vi "GAME.vi"() -> ()   [LabVIEW 2014]
panel:
  out "output 2":string[][](array[string])
  in  "8 8":string
  in  "8 7":string
  in  "8 6":string
  in  "8 5":string="7"
  in  "8 4":string
  in  "8 3":string
  in  "8 2":string
  in  "8 1":string="5"
  in  "8 0":string
  in  "7 3":string="6"
  in  "6 3":string
  in  "5 3":string="8"
  in  "4 3":string
  in  "3 2":string
  in  "2 4":string="2"
  in  "1 1":string="2"
  in  "0 8":string
  in  "0 0":string
  in  "7 8":string
  in  "7 7":string="5"
  in  "7 6":string
  in  "7 5":string
  in  "7 4":string="9"
  in  "6 8":string
  in  "6 7":string
  in  "6 6":string="8"
  in  "6 5":string
  in  "6 4":string="5"
  in  "5 8":string
  in  "5 7":string="2"
  in  "5 6":string
  in  "5 5":string
  in  "5 4":string
  in  "4 8":string="1"
  in  "4 7":string
  in  "4 6":string="3"
  in  "4 5":string
  in  "4 4":string
  in  "3 8":string
  in  "3 7":string
  in  "3 6":string
  in  "3 5":string="3"
  in  "3 4":string
  in  "3 3":string
  in  "2 8":string="5"
  in  "2 7":string
  in  "2 6":string="4"
  in  "2 5":string
  in  "1 8":string="8"
  in  "1 7":string
  in  "1 6":string
  in  "1 5":string="4"
  in  "1 4":string="3"
  in  "1 3":string
  in  "1 2":string
  in  "0 7":string="7"
  in  "0 6":string
  in  "0 5":string
  in  "0 4":string="5"
  in  "0 3":string
  in  "0 2":string
  in  "0 1":string
  in  "7 2":string
  in  "7 1":string
  in  "7 0":string="8"
  in  "6 2":string="4"
  in  "6 1":string
  in  "6 0":string="9"
  in  "5 2":string
  in  "5 1":string
  in  "5 0":string
  in  "4 2":string="9"
  in  "4 1":string
  in  "4 0":string="6"
  in  "3 1":string="7"
  in  "3 0":string
  in  "2 3":string
  in  "2 2":string="1"
  in  "2 1":string
  in  "2 0":string
  in  "1 0":string
  in  "stop":bool
  # "SUDOKU"
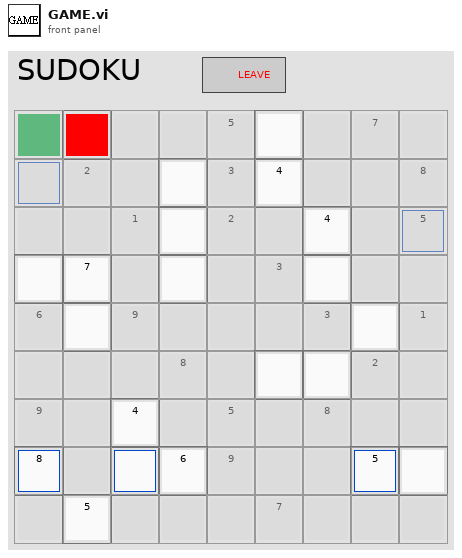
[diagram p1: front panel]
types:
  T1 = enum8{"Enabled", "Disabled", "Disabled and Grayed Out"}
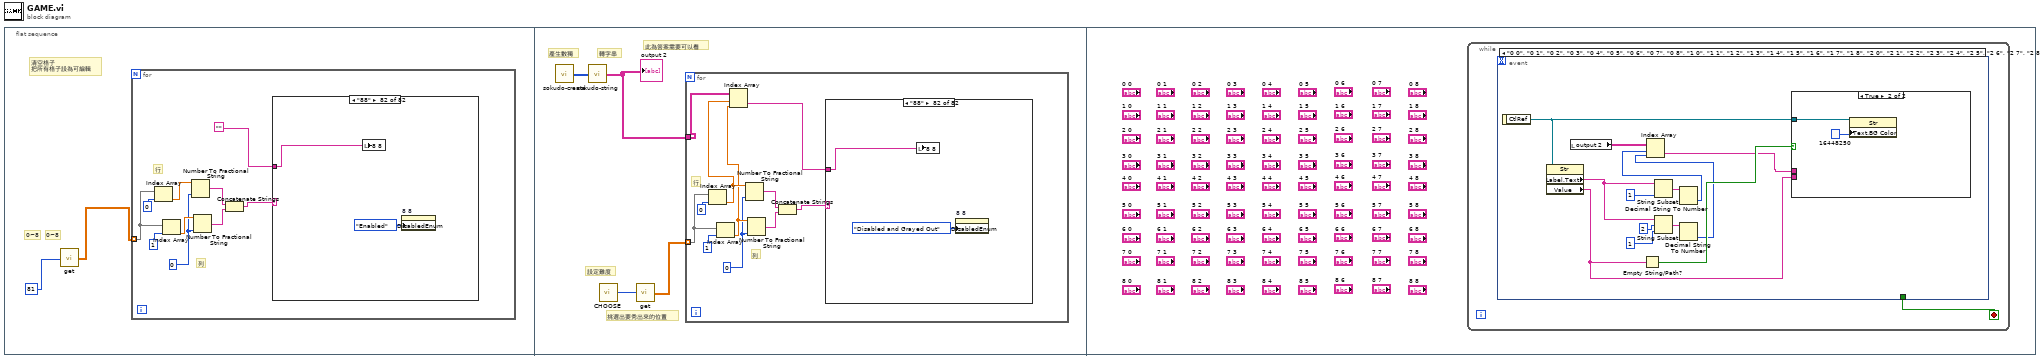
[diagram p0: block diagram]
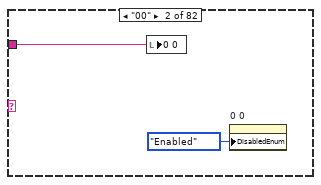
[diagram p3: hidden frame]
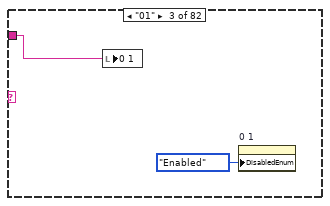
[diagram p4: hidden frame]
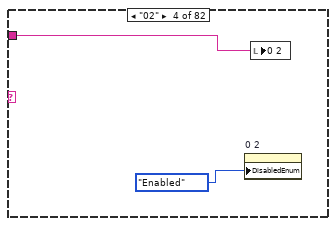
[diagram p5: hidden frame]
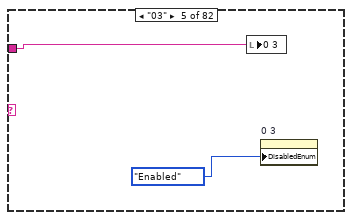
[diagram p6: hidden frame]
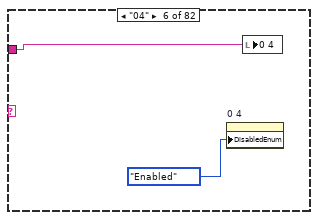
[diagram p7: hidden frame]
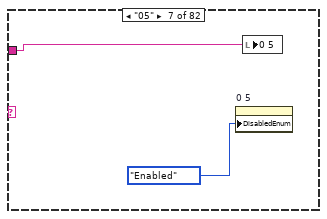
[diagram p8: hidden frame]
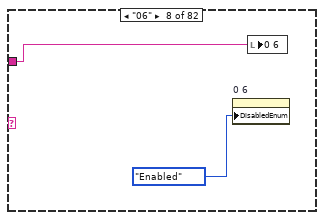
[diagram p9: hidden frame]
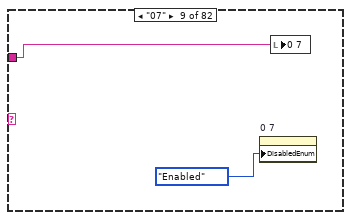
[diagram p10: hidden frame]
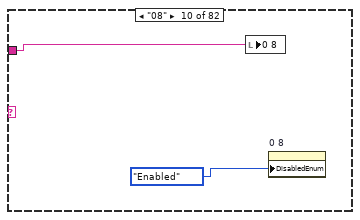
[diagram p11: hidden frame]
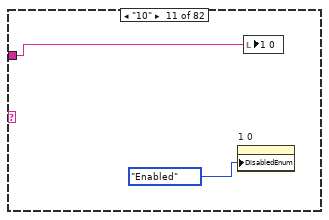
[diagram p12: hidden frame]
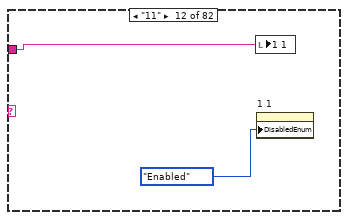
[diagram p13: hidden frame]
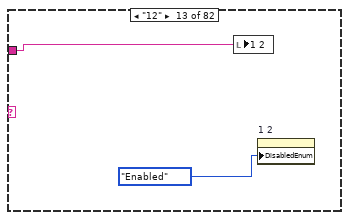
[diagram p14: hidden frame]
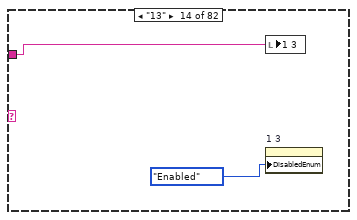
[diagram p15: hidden frame]
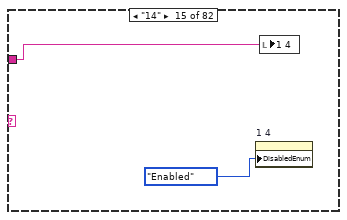
[diagram p16: hidden frame]
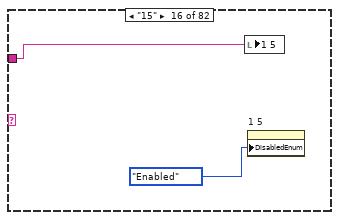
[diagram p17: hidden frame]
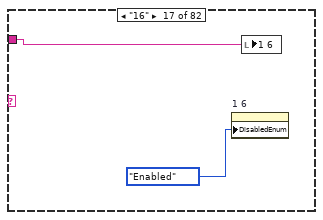
[diagram p18: hidden frame]
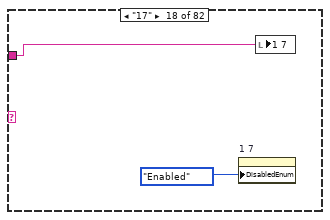
[diagram p19: hidden frame]
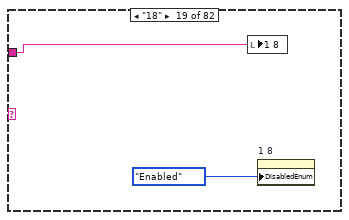
[diagram p20: hidden frame]
diagram:
  n1 = flat-sequence {
    frame #0 {
      # "0~8"
      # "0~8"
      # "清空格子\n把所有格子設為可編輯"
      n2 = call "get.vi"("Numeric 2"=81) -> ("SHOW"=w2:dbl[][])
      n3 = for {
        tunnel: w2 -> [w11] mode=indexing
        w5 = 0
        # "列"
        # "行"
        n4 = Index Array(array=w11, index=0) -> (element=w7:dbl)
        n5 = Index Array(array=w11, index=1) -> (element=w6:dbl)
        n6 = Number To Fractional String(number=w7, precision (6)=w5) -> (F-format string=w9:string)  [unwired: 2 in]
        n7 = Number To Fractional String(number=w6, precision (6)=w5) -> (F-format string=w8:string)  [unwired: 2 in]
        n8 = Concatenate Strings(w9, w8) -> (w4:string)
        n9 = case shown="\"88\"" w4 {
          tunnel: "" -> [_ w14 w16 w18 w20 w22 w24 w26 w28 w30 w32 w34 w36 w38 w40 w42 w44 w46 w48 w50 w52 w54 w56 w58 w60 w62 w64 w66 w68 w70 w72 w74 w76 w78 w80 w82 w84 w86 w88 w90 w92 w94 w96 w98 w100 w102 w104 w106 w108 w110 w112 w114 w116 w118 w120 w122 w124 w126 w128 w130 w132 w134 w136 w138 w140 w142 w144 w146 w148 w150 w152 w154 w156 w158 w160 w162 w164 w166 w168 w170 w172 w174]
          frame "False", Default {
          }
          frame "00" {
            n10 = local write "0 0"(w14) -> ()
            n11 = property on="0 0" class="Str"("DisabledEnum"=T1."Enabled" ("Disabled")) -> ()  [unwired: 2 in, 2 out]
          }
          frame "01" {
            n12 = local write "0 1"(w16) -> ()
            n13 = property on="0 1" class="Str"("DisabledEnum"=T1."Enabled" ("Disabled")) -> ()  [unwired: 2 in, 2 out]
          }
          frame "02" {
            n14 = property on="0 2" class="Str"("DisabledEnum"=T1."Enabled" ("Disabled")) -> ()  [unwired: 2 in, 2 out]
            n15 = local write "0 2"(w18) -> ()
          }
          frame "03" {
            n16 = local write "0 3"(w20) -> ()
            n17 = property on="0 3" class="Str"("DisabledEnum"=T1."Enabled" ("Disabled")) -> ()  [unwired: 2 in, 2 out]
          }
          frame "04" {
            n18 = property on="0 4" class="Str"("DisabledEnum"=T1."Enabled" ("Disabled")) -> ()  [unwired: 2 in, 2 out]
            n19 = local write "0 4"(w22) -> ()
          }
          frame "05" {
            n20 = property on="0 5" class="Str"("DisabledEnum"=T1."Enabled" ("Disabled")) -> ()  [unwired: 2 in, 2 out]
            n21 = local write "0 5"(w24) -> ()
          }
          frame "06" {
            n22 = property on="0 6" class="Str"("DisabledEnum"=T1."Enabled" ("Disabled")) -> ()  [unwired: 2 in, 2 out]
            n23 = local write "0 6"(w26) -> ()
          }
          frame "07" {
            n24 = property on="0 7" class="Str"("DisabledEnum"=T1."Enabled" ("Disabled")) -> ()  [unwired: 2 in, 2 out]
            n25 = local write "0 7"(w28) -> ()
          }
          frame "08" {
            n26 = local write "0 8"(w30) -> ()
            n27 = property on="0 8" class="Str"("DisabledEnum"=T1."Enabled" ("Disabled")) -> ()  [unwired: 2 in, 2 out]
          }
          frame "10" {
            n28 = property on="1 0" class="Str"("DisabledEnum"=T1."Enabled" ("Disabled")) -> ()  [unwired: 2 in, 2 out]
            n29 = local write "1 0"(w32) -> ()
          }
          frame "11" {
            n30 = local write "1 1"(w34) -> ()
            n31 = property on="1 1" class="Str"("DisabledEnum"=T1."Enabled" ("Disabled")) -> ()  [unwired: 2 in, 2 out]
          }
          frame "12" {
            n32 = local write "1 2"(w36) -> ()
            n33 = property on="1 2" class="Str"("DisabledEnum"=T1."Enabled" ("Disabled")) -> ()  [unwired: 2 in, 2 out]
          }
          frame "13" {
            n34 = local write "1 3"(w38) -> ()
            n35 = property on="1 3" class="Str"("DisabledEnum"=T1."Enabled" ("Disabled")) -> ()  [unwired: 2 in, 2 out]
          }
          frame "14" {
            n36 = property on="1 4" class="Str"("DisabledEnum"=T1."Enabled" ("Disabled")) -> ()  [unwired: 2 in, 2 out]
            n37 = local write "1 4"(w40) -> ()
          }
          frame "15" {
            n38 = local write "1 5"(w42) -> ()
            n39 = property on="1 5" class="Str"("DisabledEnum"=T1."Enabled" ("Disabled")) -> ()  [unwired: 2 in, 2 out]
          }
          frame "16" {
            n40 = property on="1 6" class="Str"("DisabledEnum"=T1."Enabled" ("Disabled")) -> ()  [unwired: 2 in, 2 out]
            n41 = local write "1 6"(w44) -> ()
          }
          frame "17" {
            n42 = property on="1 7" class="Str"("DisabledEnum"=T1."Enabled" ("Disabled")) -> ()  [unwired: 2 in, 2 out]
            n43 = local write "1 7"(w46) -> ()
          }
          frame "18" {
            n44 = local write "1 8"(w48) -> ()
            n45 = property on="1 8" class="Str"("DisabledEnum"=T1."Enabled" ("Disabled")) -> ()  [unwired: 2 in, 2 out]
          }
          frame "20" {
            n46 = local write "2 0"(w50) -> ()
            n47 = property on="2 0" class="Str"("DisabledEnum"=T1."Enabled" ("Disabled")) -> ()  [unwired: 2 in, 2 out]
          }
          frame "21" {
            n48 = local write "2 1"(w52) -> ()
            n49 = property on="2 1" class="Str"("DisabledEnum"=T1."Enabled" ("Disabled")) -> ()  [unwired: 2 in, 2 out]
          }
          frame "22" {
            n50 = local write "2 2"(w54) -> ()
            n51 = property on="2 2" class="Str"("DisabledEnum"=T1."Enabled" ("Disabled")) -> ()  [unwired: 2 in, 2 out]
          }
          frame "23" {
            n52 = local write "2 3"(w56) -> ()
            n53 = property on="2 3" class="Str"("DisabledEnum"=T1."Enabled" ("Disabled")) -> ()  [unwired: 2 in, 2 out]
          }
          frame "24" {
            n54 = property on="2 4" class="Str"("DisabledEnum"=T1."Enabled" ("Disabled")) -> ()  [unwired: 2 in, 2 out]
            n55 = local write "2 4"(w58) -> ()
          }
          frame "25" {
            n56 = local write "2 5"(w60) -> ()
            n57 = property on="2 5" class="Str"("DisabledEnum"=T1."Enabled" ("Disabled")) -> ()  [unwired: 2 in, 2 out]
          }
          frame "26" {
            n58 = local write "2 6"(w62) -> ()
            n59 = property on="2 6" class="Str"("DisabledEnum"=T1."Enabled" ("Disabled")) -> ()  [unwired: 2 in, 2 out]
          }
          frame "27" {
            n60 = property on="2 7" class="Str"("DisabledEnum"=T1."Enabled" ("Disabled")) -> ()  [unwired: 2 in, 2 out]
            n61 = local write "2 7"(w64) -> ()
          }
          frame "28" {
            n62 = property on="2 8" class="Str"("DisabledEnum"=T1."Enabled" ("Disabled")) -> ()  [unwired: 2 in, 2 out]
            n63 = local write "2 8"(w66) -> ()
          }
          frame "30" {
            n64 = property on="3 0" class="Str"("DisabledEnum"=T1."Enabled" ("Disabled")) -> ()  [unwired: 2 in, 2 out]
            n65 = local write "3 0"(w68) -> ()
          }
          frame "31" {
            n66 = local write "3 1"(w70) -> ()
            n67 = property on="3 1" class="Str"("DisabledEnum"=T1."Enabled" ("Disabled")) -> ()  [unwired: 2 in, 2 out]
          }
          frame "32" {
            n68 = local write "3 2"(w72) -> ()
            n69 = property on="3 2" class="Str"("DisabledEnum"=T1."Enabled" ("Disabled")) -> ()  [unwired: 2 in, 2 out]
          }
          frame "33" {
            n70 = local write "3 3"(w74) -> ()
            n71 = property on="3 3" class="Str"("DisabledEnum"=T1."Enabled" ("Disabled")) -> ()  [unwired: 2 in, 2 out]
          }
          frame "34" {
            n72 = local write "3 4"(w76) -> ()
            n73 = property on="3 4" class="Str"("DisabledEnum"=T1."Enabled" ("Disabled")) -> ()  [unwired: 2 in, 2 out]
          }
          frame "35" {
            n74 = property on="3 5" class="Str"("DisabledEnum"=T1."Enabled" ("Disabled")) -> ()  [unwired: 2 in, 2 out]
            n75 = local write "3 5"(w78) -> ()
          }
          frame "36" {
            n76 = local write "3 6"(w80) -> ()
            n77 = property on="3 6" class="Str"("DisabledEnum"=T1."Enabled" ("Disabled")) -> ()  [unwired: 2 in, 2 out]
          }
          frame "37" {
            n78 = property on="3 7" class="Str"("DisabledEnum"=T1."Enabled" ("Disabled")) -> ()  [unwired: 2 in, 2 out]
            n79 = local write "3 7"(w82) -> ()
          }
          frame "38" {
            n80 = property on="3 8" class="Str"("DisabledEnum"=T1."Enabled" ("Disabled")) -> ()  [unwired: 2 in, 2 out]
            n81 = local write "3 8"(w84) -> ()
          }
          frame "40" {
            n82 = local write "4 0"(w86) -> ()
            n83 = property on="4 0" class="Str"("DisabledEnum"=T1."Enabled" ("Disabled")) -> ()  [unwired: 2 in, 2 out]
          }
          frame "41" {
            n84 = property on="4 1" class="Str"("DisabledEnum"=T1."Enabled" ("Disabled")) -> ()  [unwired: 2 in, 2 out]
            n85 = local write "4 1"(w88) -> ()
          }
          frame "42" {
            n86 = local write "4 2"(w90) -> ()
            n87 = property on="4 2" class="Str"("DisabledEnum"=T1."Enabled" ("Disabled")) -> ()  [unwired: 2 in, 2 out]
          }
          frame "43" {
            n88 = property on="4 3" class="Str"("DisabledEnum"=T1."Enabled" ("Disabled")) -> ()  [unwired: 2 in, 2 out]
            n89 = local write "4 3"(w92) -> ()
          }
          frame "44" {
            n90 = local write "4 4"(w94) -> ()
            n91 = property on="4 4" class="Str"("DisabledEnum"=T1."Enabled" ("Disabled")) -> ()  [unwired: 2 in, 2 out]
          }
          frame "45" {
            n92 = local write "4 5"(w96) -> ()
            n93 = property on="4 5" class="Str"("DisabledEnum"=T1."Enabled" ("Disabled")) -> ()  [unwired: 2 in, 2 out]
          }
          frame "46" {
            n94 = local write "4 6"(w98) -> ()
            n95 = property on="4 6" class="Str"("DisabledEnum"=T1."Enabled" ("Disabled")) -> ()  [unwired: 2 in, 2 out]
          }
          frame "47" {
            n96 = local write "4 7"(w100) -> ()
            n97 = property on="4 7" class="Str"("DisabledEnum"=T1."Enabled" ("Disabled")) -> ()  [unwired: 2 in, 2 out]
          }
          frame "48" {
            n98 = local write "4 8"(w102) -> ()
            n99 = property on="4 8" class="Str"("DisabledEnum"=T1."Enabled" ("Disabled")) -> ()  [unwired: 2 in, 2 out]
          }
          frame "50" {
            n100 = local write "5 0"(w104) -> ()
            n101 = property on="5 0" class="Str"("DisabledEnum"=T1."Enabled" ("Disabled")) -> ()  [unwired: 2 in, 2 out]
          }
          frame "51" {
            n102 = local write "5 1"(w106) -> ()
            n103 = property on="5 1" class="Str"("DisabledEnum"=T1."Enabled" ("Disabled")) -> ()  [unwired: 2 in, 2 out]
          }
          frame "52" {
            n104 = property on="5 2" class="Str"("DisabledEnum"=T1."Enabled" ("Disabled")) -> ()  [unwired: 2 in, 2 out]
            n105 = local write "5 2"(w108) -> ()
          }
          frame "53" {
            n106 = local write "5 3"(w110) -> ()
            n107 = property on="5 3" class="Str"("DisabledEnum"=T1."Enabled" ("Disabled")) -> ()  [unwired: 2 in, 2 out]
          }
          frame "54" {
            n108 = local write "5 4"(w112) -> ()
            n109 = property on="5 4" class="Str"("DisabledEnum"=T1."Enabled" ("Disabled")) -> ()  [unwired: 2 in, 2 out]
          }
          frame "55" {
            n110 = local write "5 5"(w114) -> ()
            n111 = property on="5 5" class="Str"("DisabledEnum"=T1."Enabled" ("Disabled")) -> ()  [unwired: 2 in, 2 out]
          }
          frame "56" {
            n112 = property on="5 6" class="Str"("DisabledEnum"=T1."Enabled" ("Disabled")) -> ()  [unwired: 2 in, 2 out]
            n113 = local write "5 6"(w116) -> ()
          }
          frame "57" {
            n114 = local write "5 7"(w118) -> ()
            n115 = property on="5 7" class="Str"("DisabledEnum"=T1."Enabled" ("Disabled")) -> ()  [unwired: 2 in, 2 out]
          }
          frame "58" {
            n116 = property on="5 8" class="Str"("DisabledEnum"=T1."Enabled" ("Disabled")) -> ()  [unwired: 2 in, 2 out]
            n117 = local write "5 8"(w120) -> ()
          }
          frame "60" {
            n118 = local write "6 0"(w122) -> ()
            n119 = property on="6 0" class="Str"("DisabledEnum"=T1."Enabled" ("Disabled")) -> ()  [unwired: 2 in, 2 out]
          }
          frame "61" {
            n120 = local write "6 1"(w124) -> ()
            n121 = property on="6 1" class="Str"("DisabledEnum"=T1."Enabled" ("Disabled")) -> ()  [unwired: 2 in, 2 out]
          }
          frame "62" {
            n122 = local write "6 2"(w126) -> ()
            n123 = property on="6 2" class="Str"("DisabledEnum"=T1."Enabled" ("Disabled")) -> ()  [unwired: 2 in, 2 out]
          }
          frame "63" {
            n124 = local write "6 3"(w128) -> ()
            n125 = property on="6 3" class="Str"("DisabledEnum"=T1."Enabled" ("Disabled")) -> ()  [unwired: 2 in, 2 out]
          }
          frame "64" {
            n126 = local write "6 4"(w130) -> ()
            n127 = property on="6 4" class="Str"("DisabledEnum"=T1."Enabled" ("Disabled")) -> ()  [unwired: 2 in, 2 out]
          }
          frame "65" {
            n128 = local write "6 5"(w132) -> ()
            n129 = property on="6 5" class="Str"("DisabledEnum"=T1."Enabled" ("Disabled")) -> ()  [unwired: 2 in, 2 out]
          }
          frame "66" {
            n130 = property on="6 6" class="Str"("DisabledEnum"=T1."Enabled" ("Disabled")) -> ()  [unwired: 2 in, 2 out]
            n131 = local write "6 6"(w134) -> ()
          }
          frame "67" {
            n132 = property on="6 7" class="Str"("DisabledEnum"=T1."Enabled" ("Disabled")) -> ()  [unwired: 2 in, 2 out]
            n133 = local write "6 7"(w136) -> ()
          }
          frame "68" {
            n134 = local write "6 8"(w138) -> ()
            n135 = property on="6 8" class="Str"("DisabledEnum"=T1."Enabled" ("Disabled")) -> ()  [unwired: 2 in, 2 out]
          }
          frame "70" {
            n136 = property on="7 0" class="Str"("DisabledEnum"=T1."Enabled" ("Disabled")) -> ()  [unwired: 2 in, 2 out]
            n137 = local write "7 0"(w140) -> ()
          }
          frame "71" {
            n138 = property on="7 1" class="Str"("DisabledEnum"=T1."Enabled" ("Disabled")) -> ()  [unwired: 2 in, 2 out]
            n139 = local write "7 1"(w142) -> ()
          }
          frame "72" {
            n140 = local write "7 2"(w144) -> ()
            n141 = property on="7 2" class="Str"("DisabledEnum"=T1."Enabled" ("Disabled")) -> ()  [unwired: 2 in, 2 out]
          }
          frame "73" {
            n142 = local write "7 3"(w146) -> ()
            n143 = property on="7 3" class="Str"("DisabledEnum"=T1."Enabled" ("Disabled")) -> ()  [unwired: 2 in, 2 out]
          }
          frame "74" {
            n144 = property on="7 4" class="Str"("DisabledEnum"=T1."Enabled" ("Disabled")) -> ()  [unwired: 2 in, 2 out]
            n145 = local write "7 4"(w148) -> ()
          }
          frame "75" {
            n146 = local write "7 5"(w150) -> ()
            n147 = property on="7 5" class="Str"("DisabledEnum"=T1."Enabled" ("Disabled")) -> ()  [unwired: 2 in, 2 out]
          }
          frame "76" {
            n148 = property on="7 6" class="Str"("DisabledEnum"=T1."Enabled" ("Disabled")) -> ()  [unwired: 2 in, 2 out]
            n149 = local write "7 6"(w152) -> ()
          }
          frame "77" {
            n150 = local write "7 7"(w154) -> ()
            n151 = property on="7 7" class="Str"("DisabledEnum"=T1."Enabled" ("Disabled")) -> ()  [unwired: 2 in, 2 out]
          }
          frame "78" {
            n152 = property on="7 8" class="Str"("DisabledEnum"=T1."Enabled" ("Disabled")) -> ()  [unwired: 2 in, 2 out]
            n153 = local write "7 8"(w156) -> ()
          }
          frame "80" {
            n154 = property on="8 0" class="Str"("DisabledEnum"=T1."Enabled" ("Disabled")) -> ()  [unwired: 2 in, 2 out]
            n155 = local write "8 0"(w158) -> ()
          }
          frame "81" {
            n156 = local write "8 1"(w160) -> ()
            n157 = property on="8 1" class="Str"("DisabledEnum"=T1."Enabled" ("Disabled")) -> ()  [unwired: 2 in, 2 out]
          }
          frame "82" {
            n158 = local write "8 2"(w162) -> ()
            n159 = property on="8 2" class="Str"("DisabledEnum"=T1."Enabled" ("Disabled")) -> ()  [unwired: 2 in, 2 out]
          }
          frame "83" {
            n160 = local write "8 3"(w164) -> ()
            n161 = property on="8 3" class="Str"("DisabledEnum"=T1."Enabled" ("Disabled")) -> ()  [unwired: 2 in, 2 out]
          }
          frame "84" {
            n162 = local write "8 4"(w166) -> ()
            n163 = property on="8 4" class="Str"("DisabledEnum"=T1."Enabled" ("Disabled")) -> ()  [unwired: 2 in, 2 out]
          }
          frame "85" {
            n164 = local write "8 5"(w168) -> ()
            n165 = property on="8 5" class="Str"("DisabledEnum"=T1."Enabled" ("Disabled")) -> ()  [unwired: 2 in, 2 out]
          }
          frame "86" {
            n166 = property on="8 6" class="Str"("DisabledEnum"=T1."Enabled" ("Disabled")) -> ()  [unwired: 2 in, 2 out]
            n167 = local write "8 6"(w170) -> ()
          }
          frame "87" {
            n168 = local write "8 7"(w172) -> ()
            n169 = property on="8 7" class="Str"("DisabledEnum"=T1."Enabled" ("Disabled")) -> ()  [unwired: 2 in, 2 out]
          }
          frame "88" {
            n170 = local write "8 8"(w174) -> ()
            n171 = property on="8 8" class="Str"("DisabledEnum"=T1."Enabled" ("Disabled")) -> ()  [unwired: 2 in, 2 out]
          }
        }
      }
    }
    frame #1 {
      # "轉字串"
      # "挑選出要秀出來的位置"
      # "設定難度"
      # "產生數獨"
      # "此為答案需要可以看"
      n172 = call "sokudo-create.vi"() -> ("Sudoku"=w178:i32[][])  [unwired: 1 in]
      n173 = call "sokudo-string.vi"("Input"=w178) -> ("output"=w177:string[][])
      "output 2" <- w177
      n174 = call "CHOOSE.vi"() -> ("Numeric"=w176:i32)  [unwired: 1 in]
      n175 = call "get.vi"("Numeric 2"=w176) -> ("SHOW"=w175:dbl[][])
      n176 = for {
        tunnel: w175 -> [w188] mode=indexing
        tunnel: w177 -> [w184]
        w180 = 0
        # "列"
        # "行"
        n177 = Index Array(array=w188, index=0) -> (element=w182:dbl)
        n178 = Index Array(array=w188, index=1) -> (element=w181:dbl)
        n179 = Index Array(array=w184, index (row)=w182, index (col)=w181) -> (element=w183:string)
        n180 = Number To Fractional String(number=w182, precision (6)=w180) -> (F-format string=w186:string)  [unwired: 2 in]
        n181 = Number To Fractional String(number=w181, precision (6)=w180) -> (F-format string=w185:string)  [unwired: 2 in]
        n182 = Concatenate Strings(w186, w185) -> (w179:string)
        n183 = case shown="\"88\"" w179 {
          tunnel: w183 -> [_ w191 w193 w195 w197 w199 w201 w203 w205 w207 w209 w211 w213 w215 w217 w219 w221 w223 w225 w227 w229 w231 w233 w235 w237 w239 w241 w243 w245 w247 w249 w251 w253 w255 w257 w259 w261 w263 w265 w267 w269 w271 w273 w275 w277 w279 w281 w283 w285 w287 w289 w291 w293 w295 w297 w299 w301 w303 w305 w307 w309 w311 w313 w315 w317 w319 w321 w323 w325 w327 w329 w331 w333 w335 w337 w339 w341 w343 w345 w347 w349 w351]
          frame "False", Default {
          }
          frame "00" {
            n184 = local write "0 0"(w191) -> ()
            n185 = property on="0 0" class="Str"("DisabledEnum"=T1."Disabled and Grayed Out" ("Disabled")) -> ()  [unwired: 2 in, 2 out]
          }
          frame "01" {
            n186 = local write "0 1"(w193) -> ()
            n187 = property on="0 1" class="Str"("DisabledEnum"=T1."Disabled and Grayed Out" ("Disabled")) -> ()  [unwired: 2 in, 2 out]
          }
          frame "02" {
            n188 = property on="0 2" class="Str"("DisabledEnum"=T1."Disabled and Grayed Out" ("Disabled")) -> ()  [unwired: 2 in, 2 out]
            n189 = local write "0 2"(w195) -> ()
          }
          frame "03" {
            n190 = local write "0 3"(w197) -> ()
            n191 = property on="0 3" class="Str"("DisabledEnum"=T1."Disabled and Grayed Out" ("Disabled")) -> ()  [unwired: 2 in, 2 out]
          }
          frame "04" {
            n192 = property on="0 4" class="Str"("DisabledEnum"=T1."Disabled and Grayed Out" ("Disabled")) -> ()  [unwired: 2 in, 2 out]
            n193 = local write "0 4"(w199) -> ()
          }
          frame "05" {
            n194 = property on="0 5" class="Str"("DisabledEnum"=T1."Disabled and Grayed Out" ("Disabled")) -> ()  [unwired: 2 in, 2 out]
            n195 = local write "0 5"(w201) -> ()
          }
          frame "06" {
            n196 = property on="0 6" class="Str"("DisabledEnum"=T1."Disabled and Grayed Out" ("Disabled")) -> ()  [unwired: 2 in, 2 out]
            n197 = local write "0 6"(w203) -> ()
          }
          frame "07" {
            n198 = property on="0 7" class="Str"("DisabledEnum"=T1."Disabled and Grayed Out" ("Disabled")) -> ()  [unwired: 2 in, 2 out]
            n199 = local write "0 7"(w205) -> ()
          }
          frame "08" {
            n200 = local write "0 8"(w207) -> ()
            n201 = property on="0 8" class="Str"("DisabledEnum"=T1."Disabled and Grayed Out" ("Disabled")) -> ()  [unwired: 2 in, 2 out]
          }
          frame "10" {
            n202 = property on="1 0" class="Str"("DisabledEnum"=T1."Disabled and Grayed Out" ("Disabled")) -> ()  [unwired: 2 in, 2 out]
            n203 = local write "1 0"(w209) -> ()
          }
          frame "11" {
            n204 = local write "1 1"(w211) -> ()
            n205 = property on="1 1" class="Str"("DisabledEnum"=T1."Disabled and Grayed Out" ("Disabled")) -> ()  [unwired: 2 in, 2 out]
          }
          frame "12" {
            n206 = local write "1 2"(w213) -> ()
            n207 = property on="1 2" class="Str"("DisabledEnum"=T1."Disabled and Grayed Out" ("Disabled")) -> ()  [unwired: 2 in, 2 out]
          }
          frame "13" {
            n208 = local write "1 3"(w215) -> ()
            n209 = property on="1 3" class="Str"("DisabledEnum"=T1."Disabled and Grayed Out" ("Disabled")) -> ()  [unwired: 2 in, 2 out]
          }
          frame "14" {
            n210 = property on="1 4" class="Str"("DisabledEnum"=T1."Disabled and Grayed Out" ("Disabled")) -> ()  [unwired: 2 in, 2 out]
            n211 = local write "1 4"(w217) -> ()
          }
          frame "15" {
            n212 = local write "1 5"(w219) -> ()
            n213 = property on="1 5" class="Str"("DisabledEnum"=T1."Disabled and Grayed Out" ("Disabled")) -> ()  [unwired: 2 in, 2 out]
          }
          frame "16" {
            n214 = property on="1 6" class="Str"("DisabledEnum"=T1."Disabled and Grayed Out" ("Disabled")) -> ()  [unwired: 2 in, 2 out]
            n215 = local write "1 6"(w221) -> ()
          }
          frame "17" {
            n216 = property on="1 7" class="Str"("DisabledEnum"=T1."Disabled and Grayed Out" ("Disabled")) -> ()  [unwired: 2 in, 2 out]
            n217 = local write "1 7"(w223) -> ()
          }
          frame "18" {
            n218 = local write "1 8"(w225) -> ()
            n219 = property on="1 8" class="Str"("DisabledEnum"=T1."Disabled and Grayed Out" ("Disabled")) -> ()  [unwired: 2 in, 2 out]
          }
          frame "20" {
            n220 = local write "2 0"(w227) -> ()
            n221 = property on="2 0" class="Str"("DisabledEnum"=T1."Disabled and Grayed Out" ("Disabled")) -> ()  [unwired: 2 in, 2 out]
          }
          frame "21" {
            n222 = local write "2 1"(w229) -> ()
            n223 = property on="2 1" class="Str"("DisabledEnum"=T1."Disabled and Grayed Out" ("Disabled")) -> ()  [unwired: 2 in, 2 out]
          }
          frame "22" {
            n224 = local write "2 2"(w231) -> ()
            n225 = property on="2 2" class="Str"("DisabledEnum"=T1."Disabled and Grayed Out" ("Disabled")) -> ()  [unwired: 2 in, 2 out]
          }
          frame "23" {
            n226 = local write "2 3"(w233) -> ()
            n227 = property on="2 3" class="Str"("DisabledEnum"=T1."Disabled and Grayed Out" ("Disabled")) -> ()  [unwired: 2 in, 2 out]
          }
          frame "24" {
            n228 = property on="2 4" class="Str"("DisabledEnum"=T1."Disabled and Grayed Out" ("Disabled")) -> ()  [unwired: 2 in, 2 out]
            n229 = local write "2 4"(w235) -> ()
          }
          frame "25" {
            n230 = local write "2 5"(w237) -> ()
            n231 = property on="2 5" class="Str"("DisabledEnum"=T1."Disabled and Grayed Out" ("Disabled")) -> ()  [unwired: 2 in, 2 out]
          }
          frame "26" {
            n232 = local write "2 6"(w239) -> ()
            n233 = property on="2 6" class="Str"("DisabledEnum"=T1."Disabled and Grayed Out" ("Disabled")) -> ()  [unwired: 2 in, 2 out]
          }
          frame "27" {
            n234 = property on="2 7" class="Str"("DisabledEnum"=T1."Disabled and Grayed Out" ("Disabled")) -> ()  [unwired: 2 in, 2 out]
            n235 = local write "2 7"(w241) -> ()
          }
          frame "28" {
            n236 = property on="2 8" class="Str"("DisabledEnum"=T1."Disabled and Grayed Out" ("Disabled")) -> ()  [unwired: 2 in, 2 out]
            n237 = local write "2 8"(w243) -> ()
          }
          frame "30" {
            n238 = property on="3 0" class="Str"("DisabledEnum"=T1."Disabled and Grayed Out" ("Disabled")) -> ()  [unwired: 2 in, 2 out]
            n239 = local write "3 0"(w245) -> ()
          }
          frame "31" {
            n240 = local write "3 1"(w247) -> ()
            n241 = property on="3 1" class="Str"("DisabledEnum"=T1."Disabled and Grayed Out" ("Disabled")) -> ()  [unwired: 2 in, 2 out]
          }
          frame "32" {
            n242 = local write "3 2"(w249) -> ()
            n243 = property on="3 2" class="Str"("DisabledEnum"=T1."Disabled and Grayed Out" ("Disabled")) -> ()  [unwired: 2 in, 2 out]
          }
          frame "33" {
            n244 = local write "3 3"(w251) -> ()
            n245 = property on="3 3" class="Str"("DisabledEnum"=T1."Disabled and Grayed Out" ("Disabled")) -> ()  [unwired: 2 in, 2 out]
          }
          frame "34" {
            n246 = local write "3 4"(w253) -> ()
            n247 = property on="3 4" class="Str"("DisabledEnum"=T1."Disabled and Grayed Out" ("Disabled")) -> ()  [unwired: 2 in, 2 out]
          }
          frame "35" {
            n248 = property on="3 5" class="Str"("DisabledEnum"=T1."Disabled and Grayed Out" ("Disabled")) -> ()  [unwired: 2 in, 2 out]
            n249 = local write "3 5"(w255) -> ()
          }
          frame "36" {
            n250 = local write "3 6"(w257) -> ()
            n251 = property on="3 6" class="Str"("DisabledEnum"=T1."Disabled and Grayed Out" ("Disabled")) -> ()  [unwired: 2 in, 2 out]
          }
          frame "37" {
            n252 = property on="3 7" class="Str"("DisabledEnum"=T1."Disabled and Grayed Out" ("Disabled")) -> ()  [unwired: 2 in, 2 out]
            n253 = local write "3 7"(w259) -> ()
          }
          frame "38" {
            n254 = property on="3 8" class="Str"("DisabledEnum"=T1."Disabled and Grayed Out" ("Disabled")) -> ()  [unwired: 2 in, 2 out]
            n255 = local write "3 8"(w261) -> ()
          }
          frame "40" {
            n256 = local write "4 0"(w263) -> ()
            n257 = property on="4 0" class="Str"("DisabledEnum"=T1."Disabled and Grayed Out" ("Disabled")) -> ()  [unwired: 2 in, 2 out]
          }
          frame "41" {
            n258 = property on="4 1" class="Str"("DisabledEnum"=T1."Disabled and Grayed Out" ("Disabled")) -> ()  [unwired: 2 in, 2 out]
            n259 = local write "4 1"(w265) -> ()
          }
          frame "42" {
            n260 = local write "4 2"(w267) -> ()
            n261 = property on="4 2" class="Str"("DisabledEnum"=T1."Disabled and Grayed Out" ("Disabled")) -> ()  [unwired: 2 in, 2 out]
          }
          frame "43" {
            n262 = property on="4 3" class="Str"("DisabledEnum"=T1."Disabled and Grayed Out" ("Disabled")) -> ()  [unwired: 2 in, 2 out]
            n263 = local write "4 3"(w269) -> ()
          }
          frame "44" {
            n264 = local write "4 4"(w271) -> ()
            n265 = property on="4 4" class="Str"("DisabledEnum"=T1."Disabled and Grayed Out" ("Disabled")) -> ()  [unwired: 2 in, 2 out]
          }
          frame "45" {
            n266 = local write "4 5"(w273) -> ()
            n267 = property on="4 5" class="Str"("DisabledEnum"=T1."Disabled and Grayed Out" ("Disabled")) -> ()  [unwired: 2 in, 2 out]
          }
          frame "46" {
            n268 = local write "4 6"(w275) -> ()
            n269 = property on="4 6" class="Str"("DisabledEnum"=T1."Disabled and Grayed Out" ("Disabled")) -> ()  [unwired: 2 in, 2 out]
          }
          frame "47" {
            n270 = local write "4 7"(w277) -> ()
            n271 = property on="4 7" class="Str"("DisabledEnum"=T1."Disabled and Grayed Out" ("Disabled")) -> ()  [unwired: 2 in, 2 out]
          }
          frame "48" {
            n272 = local write "4 8"(w279) -> ()
            n273 = property on="4 8" class="Str"("DisabledEnum"=T1."Disabled and Grayed Out" ("Disabled")) -> ()  [unwired: 2 in, 2 out]
          }
          frame "50" {
            n274 = local write "5 0"(w281) -> ()
            n275 = property on="5 0" class="Str"("DisabledEnum"=T1."Disabled and Grayed Out" ("Disabled")) -> ()  [unwired: 2 in, 2 out]
          }
          frame "51" {
            n276 = local write "5 1"(w283) -> ()
            n277 = property on="5 1" class="Str"("DisabledEnum"=T1."Disabled and Grayed Out" ("Disabled")) -> ()  [unwired: 2 in, 2 out]
          }
          frame "52" {
            n278 = property on="5 2" class="Str"("DisabledEnum"=T1."Disabled and Grayed Out" ("Disabled")) -> ()  [unwired: 2 in, 2 out]
            n279 = local write "5 2"(w285) -> ()
          }
          frame "53" {
            n280 = local write "5 3"(w287) -> ()
            n281 = property on="5 3" class="Str"("DisabledEnum"=T1."Disabled and Grayed Out" ("Disabled")) -> ()  [unwired: 2 in, 2 out]
          }
          frame "54" {
            n282 = local write "5 4"(w289) -> ()
            n283 = property on="5 4" class="Str"("DisabledEnum"=T1."Disabled and Grayed Out" ("Disabled")) -> ()  [unwired: 2 in, 2 out]
          }
          frame "55" {
            n284 = local write "5 5"(w291) -> ()
            n285 = property on="5 5" class="Str"("DisabledEnum"=T1."Disabled and Grayed Out" ("Disabled")) -> ()  [unwired: 2 in, 2 out]
          }
          frame "56" {
            n286 = property on="5 6" class="Str"("DisabledEnum"=T1."Disabled and Grayed Out" ("Disabled")) -> ()  [unwired: 2 in, 2 out]
            n287 = local write "5 6"(w293) -> ()
          }
          frame "57" {
            n288 = local write "5 7"(w295) -> ()
            n289 = property on="5 7" class="Str"("DisabledEnum"=T1."Disabled and Grayed Out" ("Disabled")) -> ()  [unwired: 2 in, 2 out]
          }
          frame "58" {
            n290 = property on="5 8" class="Str"("DisabledEnum"=T1."Disabled and Grayed Out" ("Disabled")) -> ()  [unwired: 2 in, 2 out]
            n291 = local write "5 8"(w297) -> ()
          }
          frame "60" {
            n292 = local write "6 0"(w299) -> ()
            n293 = property on="6 0" class="Str"("DisabledEnum"=T1."Disabled and Grayed Out" ("Disabled")) -> ()  [unwired: 2 in, 2 out]
          }
          frame "61" {
            n294 = local write "6 1"(w301) -> ()
            n295 = property on="6 1" class="Str"("DisabledEnum"=T1."Disabled and Grayed Out" ("Disabled")) -> ()  [unwired: 2 in, 2 out]
          }
          frame "62" {
            n296 = local write "6 2"(w303) -> ()
            n297 = property on="6 2" class="Str"("DisabledEnum"=T1."Disabled and Grayed Out" ("Disabled")) -> ()  [unwired: 2 in, 2 out]
          }
          frame "63" {
            n298 = local write "6 3"(w305) -> ()
            n299 = property on="6 3" class="Str"("DisabledEnum"=T1."Disabled and Grayed Out" ("Disabled")) -> ()  [unwired: 2 in, 2 out]
          }
          frame "64" {
            n300 = local write "6 4"(w307) -> ()
            n301 = property on="6 4" class="Str"("DisabledEnum"=T1."Disabled and Grayed Out" ("Disabled")) -> ()  [unwired: 2 in, 2 out]
          }
          frame "65" {
            n302 = local write "6 5"(w309) -> ()
            n303 = property on="6 5" class="Str"("DisabledEnum"=T1."Disabled and Grayed Out" ("Disabled")) -> ()  [unwired: 2 in, 2 out]
          }
          frame "66" {
            n304 = property on="6 6" class="Str"("DisabledEnum"=T1."Disabled and Grayed Out" ("Disabled")) -> ()  [unwired: 2 in, 2 out]
            n305 = local write "6 6"(w311) -> ()
          }
          frame "67" {
            n306 = property on="6 7" class="Str"("DisabledEnum"=T1."Disabled and Grayed Out" ("Disabled")) -> ()  [unwired: 2 in, 2 out]
            n307 = local write "6 7"(w313) -> ()
          }
          frame "68" {
            n308 = local write "6 8"(w315) -> ()
            n309 = property on="6 8" class="Str"("DisabledEnum"=T1."Disabled and Grayed Out" ("Disabled")) -> ()  [unwired: 2 in, 2 out]
          }
          frame "70" {
            n310 = property on="7 0" class="Str"("DisabledEnum"=T1."Disabled and Grayed Out" ("Disabled")) -> ()  [unwired: 2 in, 2 out]
            n311 = local write "7 0"(w317) -> ()
          }
          frame "71" {
            n312 = property on="7 1" class="Str"("DisabledEnum"=T1."Disabled and Grayed Out" ("Disabled")) -> ()  [unwired: 2 in, 2 out]
            n313 = local write "7 1"(w319) -> ()
          }
          frame "72" {
            n314 = local write "7 2"(w321) -> ()
            n315 = property on="7 2" class="Str"("DisabledEnum"=T1."Disabled and Grayed Out" ("Disabled")) -> ()  [unwired: 2 in, 2 out]
          }
          frame "73" {
            n316 = local write "7 3"(w323) -> ()
            n317 = property on="7 3" class="Str"("DisabledEnum"=T1."Disabled and Grayed Out" ("Disabled")) -> ()  [unwired: 2 in, 2 out]
          }
          frame "74" {
            n318 = property on="7 4" class="Str"("DisabledEnum"=T1."Disabled and Grayed Out" ("Disabled")) -> ()  [unwired: 2 in, 2 out]
            n319 = local write "7 4"(w325) -> ()
          }
          frame "75" {
            n320 = local write "7 5"(w327) -> ()
            n321 = property on="7 5" class="Str"("DisabledEnum"=T1."Disabled and Grayed Out" ("Disabled")) -> ()  [unwired: 2 in, 2 out]
          }
          frame "76" {
            n322 = property on="7 6" class="Str"("DisabledEnum"=T1."Disabled and Grayed Out" ("Disabled")) -> ()  [unwired: 2 in, 2 out]
            n323 = local write "7 6"(w329) -> ()
          }
          frame "77" {
            n324 = local write "7 7"(w331) -> ()
            n325 = property on="7 7" class="Str"("DisabledEnum"=T1."Disabled and Grayed Out" ("Disabled")) -> ()  [unwired: 2 in, 2 out]
          }
          frame "78" {
            n326 = property on="7 8" class="Str"("DisabledEnum"=T1."Disabled and Grayed Out" ("Disabled")) -> ()  [unwired: 2 in, 2 out]
            n327 = local write "7 8"(w333) -> ()
          }
          frame "80" {
            n328 = property on="8 0" class="Str"("DisabledEnum"=T1."Disabled and Grayed Out" ("Disabled")) -> ()  [unwired: 2 in, 2 out]
            n329 = local write "8 0"(w335) -> ()
          }
          frame "81" {
            n330 = local write "8 1"(w337) -> ()
            n331 = property on="8 1" class="Str"("DisabledEnum"=T1."Disabled and Grayed Out" ("Disabled")) -> ()  [unwired: 2 in, 2 out]
          }
          frame "82" {
            n332 = local write "8 2"(w339) -> ()
            n333 = property on="8 2" class="Str"("DisabledEnum"=T1."Disabled and Grayed Out" ("Disabled")) -> ()  [unwired: 2 in, 2 out]
          }
          frame "83" {
            n334 = local write "8 3"(w341) -> ()
            n335 = property on="8 3" class="Str"("DisabledEnum"=T1."Disabled and Grayed Out" ("Disabled")) -> ()  [unwired: 2 in, 2 out]
          }
          frame "84" {
            n336 = local write "8 4"(w343) -> ()
            n337 = property on="8 4" class="Str"("DisabledEnum"=T1."Disabled and Grayed Out" ("Disabled")) -> ()  [unwired: 2 in, 2 out]
          }
          frame "85" {
            n338 = local write "8 5"(w345) -> ()
            n339 = property on="8 5" class="Str"("DisabledEnum"=T1."Disabled and Grayed Out" ("Disabled")) -> ()  [unwired: 2 in, 2 out]
          }
          frame "86" {
            n340 = property on="8 6" class="Str"("DisabledEnum"=T1."Disabled and Grayed Out" ("Disabled")) -> ()  [unwired: 2 in, 2 out]
            n341 = local write "8 6"(w347) -> ()
          }
          frame "87" {
            n342 = local write "8 7"(w349) -> ()
            n343 = property on="8 7" class="Str"("DisabledEnum"=T1."Disabled and Grayed Out" ("Disabled")) -> ()  [unwired: 2 in, 2 out]
          }
          frame "88" {
            n344 = local write "8 8"(w351) -> ()
            n345 = property on="8 8" class="Str"("DisabledEnum"=T1."Disabled and Grayed Out" ("Disabled")) -> ()  [unwired: 2 in, 2 out]
          }
        }
      }
    }
    frame #2 {
      n346 = while {
        stop <- w352 stop-if-true
        n347 = event shown="[0] \"0 0\", \"0 1\", \"0 2\", \"0 3\", \"0 4\", \"0 5\", \"0 6\", \"0 7\", \"0 8\", \"1 0\", \"1 1\", \"1 2\", \"1 3\", \"1 4\", \"1 5\", \"1 6\", \"1 7\", \"1 8\", \"2 0\", \"2 1\", \"2 2\", \"2 3\", \"2 4\", \"2 5\", \"2 6\", \"2 7\", \"2 8\", \"3 0\", \"3 1\", \"3 2\", \"3 3\", \"3 4\", \"3 5\", \"3 6\", \"3 7\", \"3 8\", \"4 0\", \"4 1\", \"4 2\", \"4 3\", \"4 4\", \"4 5\", \"4 6\", \"4 7\", \"4 8\", \"5 0\", \"5 1\", \"5 2\", \"5 3\", \"5 4\", \"5 5\", \"5 6\", \"5 7\", \"5 8\", \"6 0\", \"6 1\", \"6 2\", \"6 3\", \"6 4\", \"6 5\", \"6 6\", \"6 7\", \"6 8\", \"7 0\", \"7 1\", \"7 2\", \"7 3\", \"7 4\", \"7 5\", \"7 6\", \"7 7\", \"7 8\", \"8 0\", \"8 1\", \"8 2\", \"8 3\", \"8 4\", \"8 5\", \"8 6\", \"8 7\", \"8 8\": Value Change" {
          selector: _ -> [_ _]
          dyn-events: _ -> [_ _]
          timeout: _ -> [_ _]
          tunnel: [_ "stop"] -> w352
          event "0 0", "0 1", "0 2", "0 3", "0 4", "0 5", "0 6", "0 7", "0 8", "1 0", "1 1", "1 2", "1 3", "1 4", "1 5", "1 6", "1 7", "1 8", "2 0", "2 1", "2 2", "2 3", "2 4", "2 5", "2 6", "2 7", "2 8", "3 0", "3 1", "3 2", "3 3", "3 4", "3 5", "3 6", "3 7", "3 8", "4 0", "4 1", "4 2", "4 3", "4 4", "4 5", "4 6", "4 7", "4 8", "5 0", "5 1", "5 2", "5 3", "5 4", "5 5", "5 6", "5 7", "5 8", "6 0", "6 1", "6 2", "6 3", "6 4", "6 5", "6 6", "6 7", "6 8", "7 0", "7 1", "7 2", "7 3", "7 4", "7 5", "7 6", "7 7", "7 8", "8 0", "8 1", "8 2", "8 3", "8 4", "8 5", "8 6", "8 7", "8 8": Value Change {
            n348 = event-data() -> ("CtlRef"=w353:refnum<vi>)  [unwired: 1 in]
            n349 = property class="Str"(reference=w353) -> ("Label.Text"=w355:string, "Value"=w359:string)  [unwired: 1 in, 2 out]
            n350 = local read "output 2"() -> (w358:string[][])
            n351 = Empty String/Path?(string/path=w359) -> (empty?=w360:bool)
            n352 = String Subset(string=w355, length (rest)=1 ("length (rest)")) -> (substring=w362:string)  [unwired: 1 in]
            n353 = String Subset(string=w355, offset (0)=2, length (rest)=1 ("length (rest)")) -> (substring=w361:string)
            n354 = Decimal String To Number(string=w362) -> (number=w357:i32)  [unwired: 2 in, 1 out]
            n355 = Decimal String To Number(string=w361) -> (number=w356:i32)  [unwired: 2 in, 1 out]
            n356 = Index Array(array=w358, index (row)=w357, index (col)=w356) -> (element=w354:string)
            n357 = case shown="True" w360 {
              tunnel: w359 -> [w369 _]
              tunnel: w353 -> [w368 w374]
              tunnel: w354 -> [w366 _]
              frame False {
                n358 = Equal?(x=w366, y=w369) -> (x = y?=w367:bool)
                n359 = case shown="False" w367 {
                  tunnel: w368 -> [w370 w372]
                  frame True {
                    n360 = property on="Property Node" class="Str"(reference=w370, "Text.BG Color"=u32 46145 ("Color Box")) -> ()  [unwired: 1 in, 2 out]
                  }
                  frame False {
                    n361 = property on="Property Node" class="Str"(reference=w372, "Text.BG Color"=u32 16711680 ("Color Box")) -> ()  [unwired: 1 in, 2 out]
                  }
                }
              }
              frame True {
                n362 = property on="Property Node" class="Str"(reference=w374, "Text.BG Color"=u32 16448250 ("Color Box")) -> ()  [unwired: 1 in, 2 out]
              }
            }
          }
          event "stop": Value Change {
            n363 = event-data() -> ()  [unwired: 1 in, 3 out]
          }
        }
      }
    }
  }
